vi "Ping an IP address and show indication.vi"(4 "SITE ID":string, 6 "recipients":string[](array[string]), 7 "Responce Lite Reference":refnum<vi>, 8 "error in (no error)":errorcluster, 9 "Email Notification Cluster":T1, 10 "AddressNode 1":string, 11 "Ping Site":bool) -> (0 "error out":errorcluster)   [LabVIEW 2011]
uses:
  Controls/Ping address and email notify.ctl
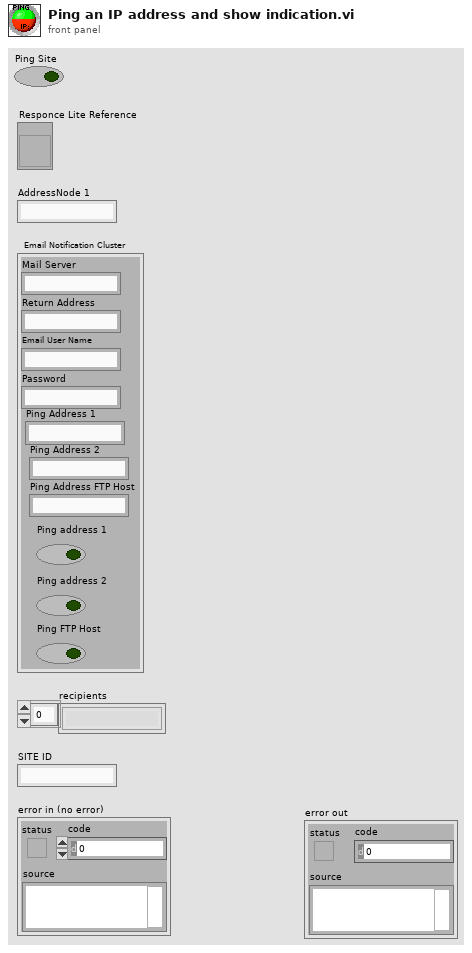
[diagram p1: front panel]
types:
  T1 = typedef "Ping address and email notify.ctl" = cluster{"Mail Server":string, "Return Address":string, "Email User Name":string, "Password":string, "Ping Address 1":string, "Ping Address 2":string, "Ping Address FTP Host":string, "Ping address 1":bool, "Ping address 2":bool, "Ping FTP Host":bool}
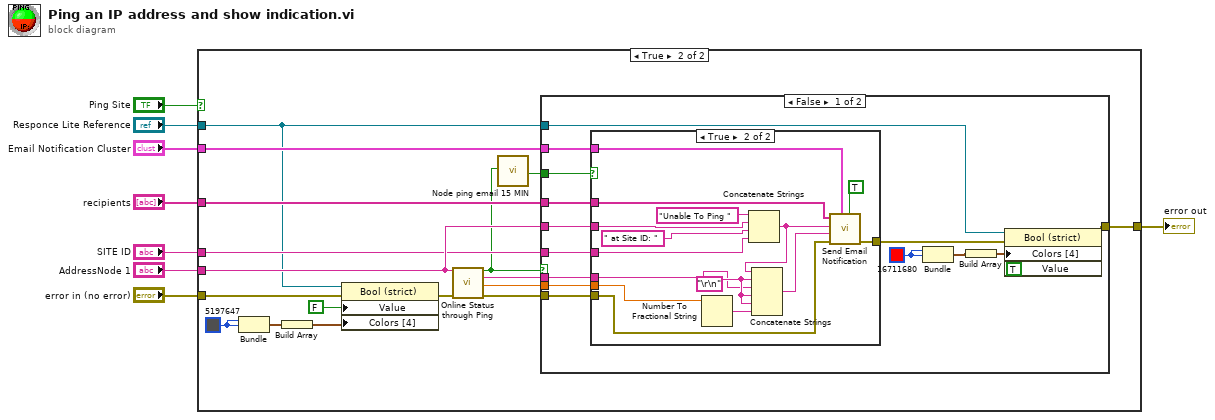
[diagram p0: block diagram]
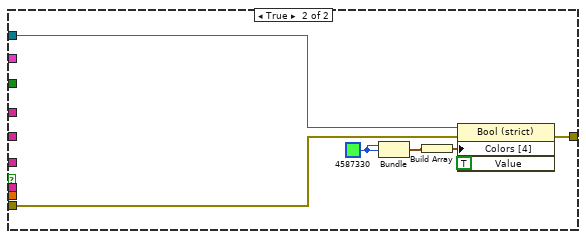
[diagram p4: hidden frame]
diagram:
  n1 = case shown="True" "Ping Site" {
    tunnel: "AddressNode 1" -> [_ w24]
    tunnel: [w9 w23] -> w2
    tunnel: "recipients" -> [_ w22]
    tunnel: "error in (no error)" -> [w9 w12]
    tunnel: "SITE ID" -> [_ w21]
    tunnel: "Email Notification Cluster" -> [_ w20]
    tunnel: "Responce Lite Reference" -> [_ w14]
    frame False {
    }
    frame True {
      w15 = u32 5197647 ("Color Box")
      n2 = Bundle("Color Box"=w15, "Color Box"=w15) -> (w16:cluster{"Color Box":u32, "Color Box":u32})  [unwired: 1 in]
      n3 = Build Array(w16) -> (w10:cluster{"Color Box":u32, "Color Box":u32}[])
      n4 = property class="Bool (strict)"(reference=w14, error in=w12, "Value"=FALSE ("Response 1"), "Colors [4]"=w10) -> (error out=w13:errorcluster)  [unwired: 1 out]
      n5 = call "Online Status through Ping.vi"("AddressToPing"=w24, "error in (no error)"=w13) -> ("Connection?"=w18:bool, "Standard Output"=w26:string, "% Recieved"=w25:dbl, "error out"=w17:errorcluster)  [unwired: 9 in, 1 out]
      n6 = call "Node ping email 15 MIN"("Reset"=w18) -> ("Time has Elapsed"=w19:bool)  [unwired: 11 in, 7 out]
      n7 = case shown="False" w18 {
        tunnel: w26 -> [w41 _]
        tunnel: w25 -> [w40 _]
        tunnel: w22 -> [w39 _]
        tunnel: w24 -> [w38 _]
        tunnel: w21 -> [w34 _]
        tunnel: w17 -> [w33 w61]
        tunnel: [w29 w60] -> w23
        tunnel: w20 -> [w32 _]
        tunnel: w19 -> [w31 _]
        tunnel: w14 -> [w27 w58]
        frame False {
          w36 = u32 16711680 ("Color Box")
          n8 = case shown="True" w31 {
            tunnel: w41 -> [_ w52]
            tunnel: w40 -> [_ w54]
            tunnel: w39 -> [_ w46]
            tunnel: w38 -> [_ w53]
            tunnel: w34 -> [_ w50]
            tunnel: w33 -> [w42 w43]
            tunnel: [w42 w49] -> w30
            tunnel: w32 -> [_ w47]
            frame False {
            }
            frame True {
              w56 = "\r\n"
              n9 = Number To Fractional String(number=w54) -> (F-format string=w55:string)  [unwired: 3 in]
              n10 = Concatenate Strings("Unable To Ping " ("subject ([No Subject])"), w53, " at Site ID: " ("string"), w50) -> (w45:string)
              n11 = Concatenate Strings(w45, w56, w52, w56, w56, w55) -> (w44:string)
              n12 = call "Send Email Notification.vi"("Send Email Notification"=TRUE, "Email Notification Cluster (in)"=w47, "Error IN"=w43, "message"=w44, "Email Subject"=w45, "recipients"=w46) -> ("error out"=w49:errorcluster)  [unwired: 5 in]
            }
          }
          n13 = Bundle("Color Box"=w36, "Color Box"=w36) -> (w35:cluster{"Color Box":u32, "Color Box":u32})  [unwired: 1 in]
          n14 = Build Array(w35) -> (w37:cluster{"Color Box":u32, "Color Box":u32}[])
          n15 = property on="Property Node" class="Bool (strict)"(reference=w27, error in=w30, "Colors [4]"=w37, "Value"=TRUE ("Node Responding")) -> (error out=w29:errorcluster)  [unwired: 1 out]
        }
        frame True {
          w63 = u32 4587330 ("Color Box")
          n16 = Bundle("Color Box"=w63, "Color Box"=w63) -> (w64:cluster{"Color Box":u32, "Color Box":u32})  [unwired: 1 in]
          n17 = Build Array(w64) -> (w62:cluster{"Color Box":u32, "Color Box":u32}[])
          n18 = property on="Property Node" class="Bool (strict)"(reference=w58, error in=w61, "Colors [4]"=w62, "Value"=TRUE ("Response 1")) -> (error out=w60:errorcluster)  [unwired: 1 out]
        }
      }
    }
  }
  "error out" <- w2
